vi "LV to DAT.vi"(6 "append to file? (new file:F)":bool, 7 "path":path, 8 "wavenames (.Vx, etc)":string[](array[string]), 9 "Data":dbl[](array[numeric]), 10 "Comments":string, 11 "filename":string) -> (3 "new file path":path)   [LabVIEW 2016, in "LVtoITX.lvclass"]
uses:
  LVtoITX.lvclass
  <vilib>/Utility/file.llb/Write Delimited Spreadsheet (string).vi
panel:
  out "appended array":string[][](array[string])
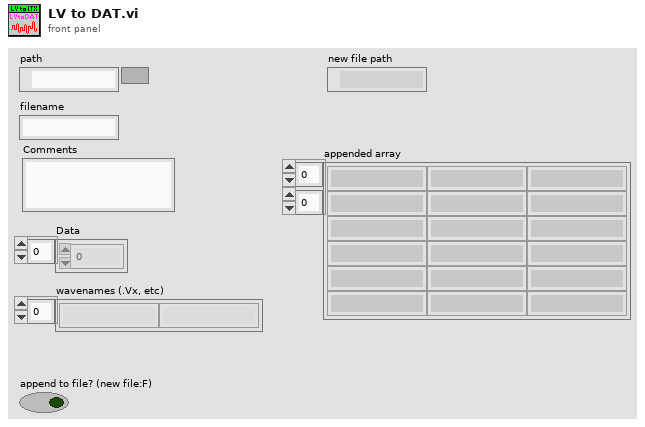
[diagram p1: front panel]
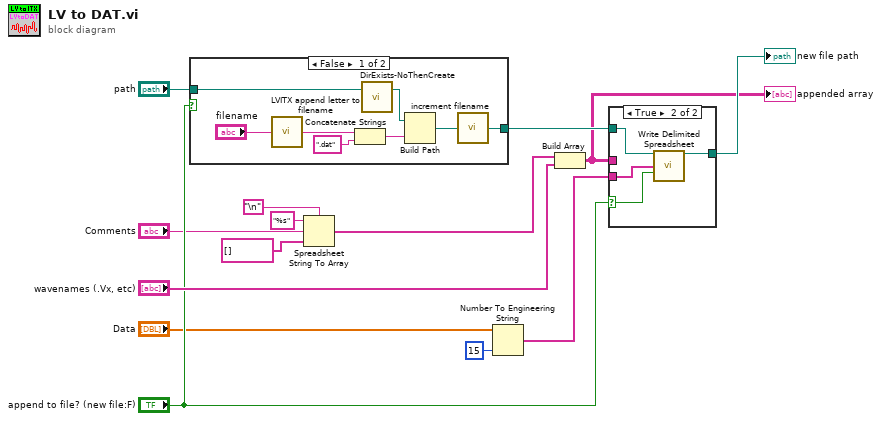
[diagram p0: block diagram]
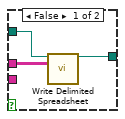
[diagram p3: hidden frame]
diagram:
  n1 = case shown="False" "append to file? (new file:F)" {
    tunnel: [w22 w23] -> w14
    tunnel: "path" -> [w20 w23]
    frame False {
      n2 = call "LVITX append letter to filename.vi"("string in"="filename") -> ("string out"=w15:string)
      n3 = Concatenate Strings(w15, ".dat" ("string")) -> (w16:string)
      n4 = call <userlib>:"DirExists-NoThenCreate.vi"("path"=w20) -> ("created path"=w17:path)  [unwired: 1 in, 1 out]
      n5 = Build Path(base path=w17, name or relative path=w16) -> (appended path=w18:path)
      n6 = call <userlib>:"increment filename.vi"("path"=w18) -> ("modified path"=w22:path)
    }
    frame True {
    }
  }
  n7 = Spreadsheet String To Array(delimiter (Tab)="\n", format string="%s", spreadsheet string="Comments", array type (2D Dbl)=string[] []) -> (array=w8:string[])
  n8 = Number To Engineering String(2:i16 15 ("precision (6)"), 4:"Data") -> (0:w2:string[])  [unwired: 2 out]
  n9 = Build Array(w8, "wavenames (.Vx, etc)") -> (w1:string[][])
  "appended array" <- w1
  n10 = case shown="True" "append to file? (new file:F)" {
    selector: "append to file? (new file:F)" -> [_ w28]
    tunnel: w1 -> [w24 _]
    tunnel: [w26 w30] -> w12
    tunnel: w2 -> [_ w27]
    tunnel: w14 -> [w25 w29]
    frame False {
      n11 = call-poly <vilib>:"Write Delimited Spreadsheet.vi"("file path (dialog if empty)"=w25, "2D data"=w24) -> ("new file path (Not A Path if cancelled)"=w26:path)  [unwired: 12 in, 1 out]
    }
    frame True {
      n12 = call-poly <vilib>:"Write Delimited Spreadsheet.vi"("file path (dialog if empty)"=w29, "1D data"=w27, "append to file? (new file:F)"=w28) -> ("new file path (Not A Path if cancelled)"=w30:path)  [unwired: 11 in, 1 out]
    }
  }
  "new file path" <- w12
